vi "Perform_large_file_Analysis.vi"(7 "error in":errorcluster) -> (2 "Wvfm":waveform(dbl)[](array[waveform]), 3 "Filtered Nb of Events":i32, 5 "Total Nb of Events":dbl)   [LabVIEW 2019]
uses:
  <vilib>/Utility/error.llb/DialogType.ctl
  ESA_Data_Analysis_Global_VIs.vi
  SiPM_Tests_Global_Var.vi
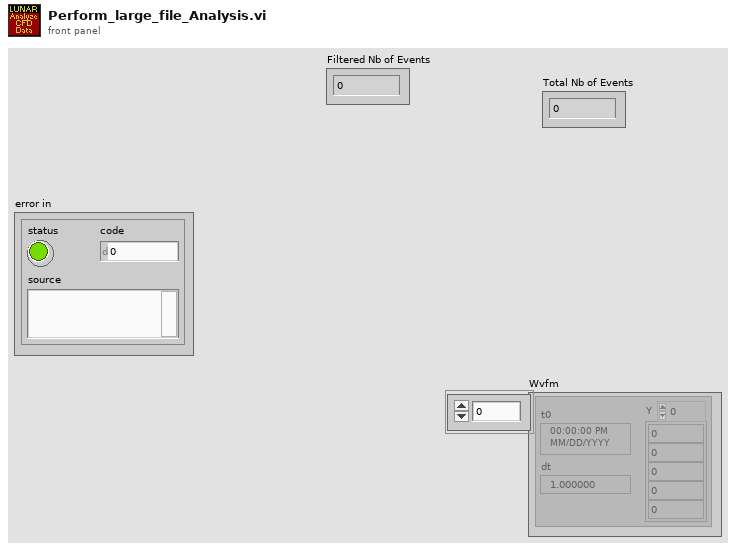
[diagram p1: front panel]
types:
  T1 = typedef "DialogType.ctl" = u16
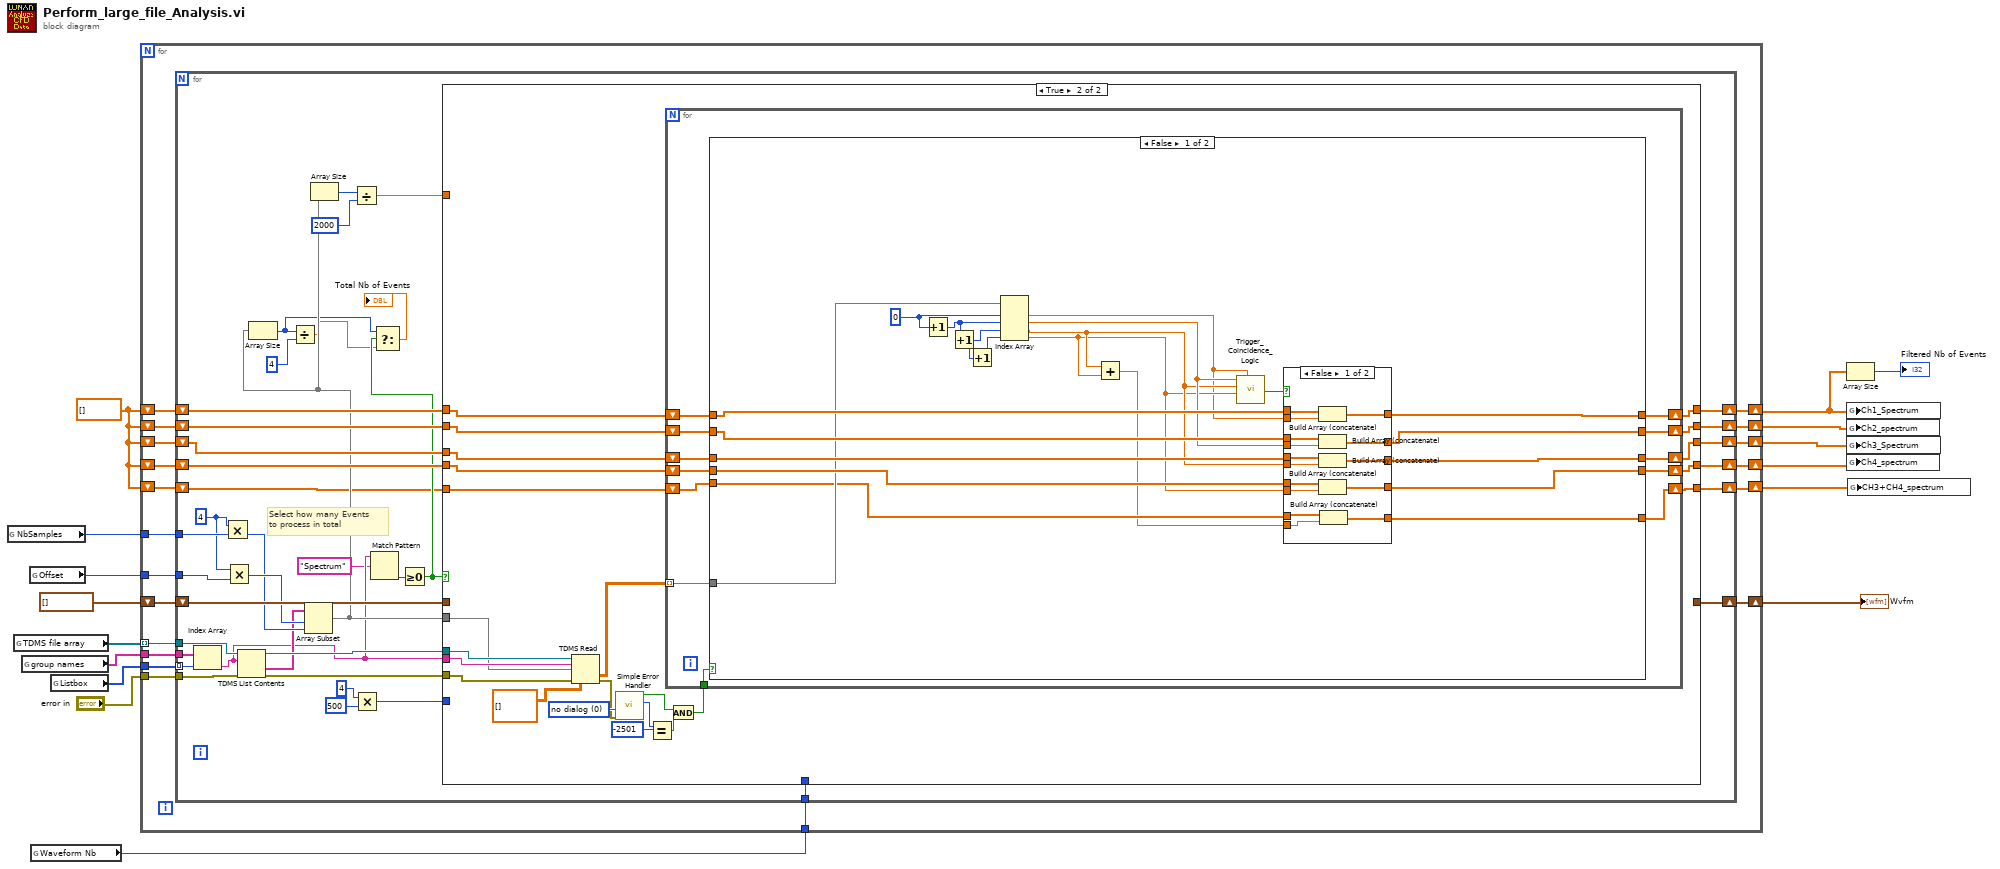
[diagram p0: block diagram]
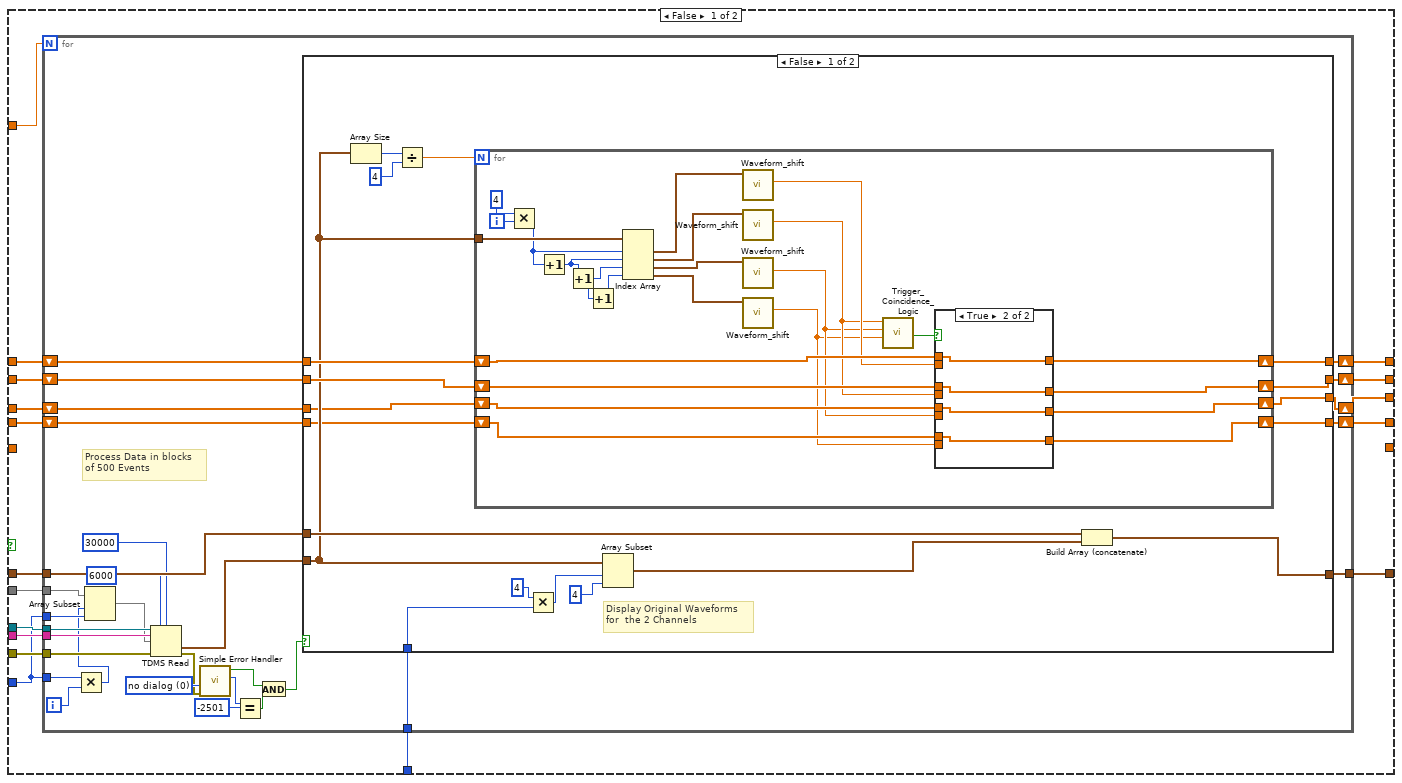
[diagram p2: hidden frame]
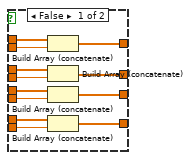
[diagram p3: hidden frame]
diagram:
  w2 = dbl[] []
  n1 = global read "SiPM_Tests_Global_Var.vi" "NbSamples"() -> (w9:i64)
  n2 = global read "SiPM_Tests_Global_Var.vi" "TDMS file array"() -> (w13:refnum<k34>[])
  n3 = global read "ESA_Data_Analysis_Global_VIs.vi" "group names"() -> (w16:string[])
  n4 = global read "SiPM_Tests_Global_Var.vi" "Offset"() -> (w11:i64)
  n5 = global read "SiPM_Tests_Global_Var.vi" "Waveform Nb"() -> (w8:u16)
  n6 = global read "ESA_Data_Analysis_Global_VIs.vi" "Listbox"() -> (w15:i32[])
  n7 = for {
    tunnel: w13 -> [w35] mode=indexing
    tunnel: w16 -> [w34]
    tunnel: w15 -> [w33]
    tunnel: "error in" -> [w32]
    tunnel: w11 -> [w30]
    shift-right: [w31] -> w12
    shift-left: waveform(dbl)[] [] -> [w29]
    shift-right: [w25] -> w7
    shift-left: w2 -> [w28]
    shift-right: [w26] -> w4
    shift-left: w2 -> [w27]
    tunnel: w9 -> [w24]
    tunnel: w8 -> [w23]
    shift-right: [w20] -> w6
    shift-left: w2 -> [w22]
    shift-right: [w19] -> w5
    shift-left: w2 -> [w21]
    shift-right: [w17] -> w1
    shift-left: w2 -> [w18]
    n8 = for {
      tunnel: w35 -> [w75]
      tunnel: w34 -> [w74]
      tunnel: w33 -> [w73] mode=indexing
      tunnel: w32 -> [w72]
      tunnel: w30 -> [w62]
      shift-right: [w69] -> w31
      shift-left: w29 -> [w68]
      shift-right: [w64] -> w25
      shift-left: w28 -> [w67]
      shift-right: [w65] -> w26
      shift-left: w27 -> [w66]
      tunnel: w24 -> [w61]
      tunnel: w23 -> [w63]
      shift-right: [w57] -> w20
      shift-left: w22 -> [w59]
      shift-right: [w56] -> w19
      shift-left: w21 -> [w58]
      shift-right: [w36] -> w17
      shift-left: w18 -> [w37]
      w60 = i64 4 ("x")
      # "Select how many Events \nto process in total"
      n9 = Index Array(array=w74, index=w73) -> (element=w44:string)
      n10 = Multiply(x=w60, y=w61) -> (x*y=w54:i64)
      n11 = Multiply(x=w60, y=w62) -> (x*y=w55:i64)
      n12 = TDMS List Contents(4:w72, 6:w44, 7:w75) -> (0:w70:errorcluster, 1:w53:string[], 3:w71:refnum<k34>)  [unwired: 1 out]
      n13 = Array Subset(array=w53, index=w55, length=w54) -> (w45:string[])
      n14 = Array Size(array=w45) -> (size(s)=w40:i32)
      n15 = Divide(x=w40, y=4) -> (x/y=w39:dbl)
      n16 = Array Size(array=w45) -> (size(s)=w48:i32)
      n17 = Divide(x=w48, y=2000) -> (x/y=w47:dbl)
      n18 = Multiply(x=i64 4, y=i64 500) -> (x*y=w50:i64)
      n19 = Match Pattern(string=w44, regular expression="Spectrum") -> (offset past match=w42:i32)  [unwired: 1 in, 3 out]
      n20 = Greater Or Equal To 0?(x=w42) -> (x >= 0?=w41:bool)
      n21 = Select(t=w40, s=w41, f=w39) -> (s? t:f=→"Total Nb of Events":dbl)
      n22 = case shown="True" w41 {
        tunnel: w71 -> [w92 w207]
        tunnel: w44 -> [w91 w208]
        tunnel: w70 -> [w90 w209]
        tunnel: [w89 _] -> w69
        tunnel: w68 -> [w88 _]
        tunnel: w67 -> [w87 w197]
        tunnel: w66 -> [w86 w198]
        tunnel: [w85 w194] -> w65
        tunnel: [w84 w193] -> w64
        tunnel: w63 -> [w83 _]
        tunnel: w59 -> [w82 w196]
        tunnel: w58 -> [w81 w195]
        tunnel: [w80 w192] -> w57
        tunnel: [w79 w191] -> w56
        tunnel: w50 -> [w78 _]
        tunnel: w47 -> [w77 _]
        tunnel: w45 -> [w76 w190]
        tunnel: w37 -> [_ w188]
        tunnel: [_ w187] -> w36
        frame False {
          n23 = for {
            N: w77 -> [_]
            tunnel: w92 -> [w122]
            tunnel: w91 -> [w121]
            tunnel: w90 -> [w118]
            tunnel: [w117] -> w89
            tunnel: w88 -> [w116]
            tunnel: w83 -> [w106]
            tunnel: w76 -> [w100]
            shift-right: [w108] -> w85
            shift-left: w86 -> [w109]
            shift-right: [w107] -> w84
            shift-left: w87 -> [w110]
            shift-right: [w103] -> w80
            shift-left: w82 -> [w105]
            shift-right: [w102] -> w79
            shift-left: w81 -> [w104]
            tunnel: w78 -> [w98]
            tunnel: w78 -> [w96]
            i -> [w97]
            w120 = T1 0 items=["no dialog", "OK message", "continue or stop message", "OK message + warnings", "continue/stop + warnings"] ("type of dialog (OK msg:1)")
            # "Process Data in blocks \nof 500 Events"
            n24 = Multiply(x=w96, y=w97) -> (x*y=w95:i64)
            n25 = Array Subset(array=w100, index=w95, length=w98) -> (w99:string[])
            n26 = TDMS Read(0:w122, 1:i64 6000 ("offset (0)"), 2:i64 30000 ("count (-1: all)"), 5:w121, 7:w99, 11:w118) -> (10:w101:waveform(dbl)[], 15:w119:errorcluster)  [unwired: 2 in, 4 out]
            n27 = call <vilib>:"Simple Error Handler.vi"("type of dialog (OK msg:1)"=w120, "error in (no error)"=w119) -> ("error?"=w114:bool, "code out"=w113:i32)  [unwired: 3 in, 3 out]
            n28 = Equal?(x=w113, y=-2501) -> (x = y?=w111:bool)
            n29 = And(x=w114, y=w111) -> (x .and. y?=w115:bool)
            n30 = case shown="False" w115 {
              tunnel: w101 -> [w127 _]
              tunnel: [w140 w186] -> w117
              tunnel: w116 -> [w139 w186]
              tunnel: w110 -> [w135 w184]
              tunnel: w109 -> [w134 w185]
              tunnel: [w133 w185] -> w108
              tunnel: [w132 w184] -> w107
              tunnel: w106 -> [w128 _]
              tunnel: w105 -> [w126 w183]
              tunnel: w104 -> [w125 w182]
              tunnel: [w124 w183] -> w103
              tunnel: [w123 w182] -> w102
              frame False {
                # "Display Original Waveforms\nfor  the 2 Channels"
                n31 = Array Size(array=w127) -> (size(s)=w138:i32)
                n32 = Divide(x=w138, y=4) -> (x/y=w136:dbl)
                n33 = for {
                  N: w136 -> [_]
                  tunnel: w127 -> [w165]
                  shift-right: [w152] -> w133
                  shift-left: w134 -> [w153]
                  shift-right: [w150] -> w132
                  shift-left: w135 -> [w160]
                  shift-right: [w148] -> w124
                  shift-left: w126 -> [w149]
                  shift-right: [w147] -> w123
                  shift-left: w125 -> [w146]
                  i -> [w159]
                  n34 = Multiply(x=4, y=w159) -> (x*y=w163:i32)
                  n35 = Increment(x=w163) -> (x+1=w158:i32)
                  n36 = Increment(x=w158) -> (x+1=w156:i32)
                  n37 = Increment(x=w156) -> (x+1=w157:i32)
                  n38 = Index Array(array=w165, index #1=w163, index #2=w158, index #3=w156, index #4=w157) -> (element #1=w162:waveform(dbl), element #2=w161:waveform(dbl), element #3=w155:waveform(dbl), element #4=w154:waveform(dbl))
                  n39 = call "Waveform_shift.vi"("Waveform_in"=w162) -> ("Peak Value"=w151:dbl)  [unwired: 9 in]
                  n40 = call "Waveform_shift.vi"("Waveform_in"=w161) -> ("Peak Value"=w144:dbl)  [unwired: 9 in]
                  n41 = call "Waveform_shift.vi"("Waveform_in"=w155) -> ("Peak Value"=w143:dbl)  [unwired: 9 in]
                  n42 = call "Waveform_shift.vi"("Waveform_in"=w154) -> ("Peak Value"=w142:dbl)  [unwired: 9 in]
                  n43 = call "Trigger_Coincidence_Logic.vi"("Peak_ch4"=w142, "Peak_ch3"=w143, "Peak_ch2"=w144) -> ("Filter-out"=w145:bool)  [unwired: 8 in]
                  n44 = case shown="True" w145 {
                    tunnel: w160 -> [w177 w180]
                    tunnel: w144 -> [w176 _]
                    tunnel: w153 -> [w175 w181]
                    tunnel: [w174 w181] -> w152
                    tunnel: w151 -> [w173 _]
                    tunnel: [w172 w180] -> w150
                    tunnel: w149 -> [w171 w179]
                    tunnel: w143 -> [w170 _]
                    tunnel: [w169 w179] -> w148
                    tunnel: [w168 w178] -> w147
                    tunnel: w146 -> [w167 w178]
                    tunnel: w142 -> [w166 _]
                    frame False {
                      n45 = Build Array (concatenate)(w175, w173) -> (w174:dbl[])
                      n46 = Build Array (concatenate)(w177, w176) -> (w172:dbl[])
                      n47 = Build Array (concatenate)(w171, w170) -> (w169:dbl[])
                      n48 = Build Array (concatenate)(w167, w166) -> (w168:dbl[])
                    }
                    frame True {
                    }
                  }
                }
                n49 = Multiply(x=4, y=w128) -> (x*y=w131:i32)
                n50 = Array Subset(array=w127, index=w131, length=4) -> (w141:waveform(dbl)[])
                n51 = Build Array (concatenate)(w139, w141) -> (w140:waveform(dbl)[])
              }
              frame True {
              }
            }
          }
        }
        frame True {
          w206 = T1 0 items=["no dialog", "OK message", "continue or stop message", "OK message + warnings", "continue/stop + warnings"] ("type of dialog (OK msg:1)")
          n52 = TDMS Read(0:w207, 5:w208, 7:w190, 11:w209, 12:dbl[][] []) -> (10:w199:dbl[][], 15:w205:errorcluster)  [unwired: 3 in, 4 out]
          n53 = call <vilib>:"Simple Error Handler.vi"("type of dialog (OK msg:1)"=w206, "error in (no error)"=w205) -> ("error?"=w203:bool, "code out"=w202:i32)  [unwired: 3 in, 3 out]
          n54 = Equal?(x=w202, y=-2501) -> (x = y?=w200:bool)
          n55 = And(x=w203, y=w200) -> (x .and. y?=w204:bool)
          n56 = for {
            tunnel: w204 -> [w221]
            tunnel: w199 -> [w220] mode=indexing
            shift-right: [w212] -> w191
            shift-left: w195 -> [w216]
            shift-right: [w213] -> w192
            shift-left: w196 -> [w217]
            shift-right: [w214] -> w193
            shift-left: w197 -> [w218]
            shift-right: [w215] -> w194
            shift-left: w198 -> [w219]
            shift-right: [w210] -> w187
            shift-left: w188 -> [w211]
            n57 = case shown="False" w221 {
              tunnel: w218 -> [w242 w266]
              tunnel: w219 -> [w241 w267]
              tunnel: [w240 w267] -> w215
              tunnel: [w239 w266] -> w214
              tunnel: w217 -> [w238 w265]
              tunnel: w216 -> [w237 w264]
              tunnel: [w236 w265] -> w213
              tunnel: [w235 w264] -> w212
              tunnel: w220 -> [w234 _]
              tunnel: w211 -> [w225 w263]
              tunnel: [w223 w263] -> w210
              frame False {
                w228 = 0 ("x")
                n58 = Increment(x=w228) -> (x+1=w233:i32)
                n59 = Increment(x=w233) -> (x+1=w231:i32)
                n60 = Increment(x=w231) -> (x+1=w232:i32)
                n61 = Index Array(array=w234, index #1=w228, index #2=w233, index #3=w231, index #4=w232) -> (element #1=w222:dbl, element #2=w229:dbl, element #3=w227:dbl, element #4=w226:dbl)
                n62 = Add(x=w227, y=w226) -> (x+y=w224:dbl)
                n63 = call "Trigger_Coincidence_Logic.vi"("Peak_ch1"=w222, "Peak_ch4"=w226, "Peak_ch3"=w227, "Peak_ch2"=w229) -> ("Filter-out"=w230:bool)  [unwired: 7 in]
                n64 = case shown="False" w230 {
                  tunnel: w242 -> [w257 w261]
                  tunnel: w229 -> [w256 _]
                  tunnel: w241 -> [w255 w262]
                  tunnel: [w254 w262] -> w240
                  tunnel: w222 -> [w253 _]
                  tunnel: [w252 w261] -> w239
                  tunnel: w238 -> [w251 w260]
                  tunnel: w227 -> [w250 _]
                  tunnel: [w249 w260] -> w236
                  tunnel: [w248 w259] -> w235
                  tunnel: w237 -> [w247 w259]
                  tunnel: w226 -> [w246 _]
                  tunnel: w225 -> [w245 w258]
                  tunnel: w224 -> [w244 _]
                  tunnel: [w243 w258] -> w223
                  frame False {
                    n65 = Build Array (concatenate)(w255, w253) -> (w254:dbl[])
                    n66 = Build Array (concatenate)(w257, w256) -> (w252:dbl[])
                    n67 = Build Array (concatenate)(w251, w250) -> (w249:dbl[])
                    n68 = Build Array (concatenate)(w247, w246) -> (w248:dbl[])
                    n69 = Build Array (concatenate)(w245, w244) -> (w243:dbl[])
                  }
                  frame True {
                  }
                }
              }
              frame True {
              }
            }
          }
        }
      }
    }
  }
  "Wvfm" <- w12
  n70 = Array Size(array=w4) -> (size(s)=→"Filtered Nb of Events":i32)
  n71 = global write "SiPM_Tests_Global_Var.vi" "Ch1_Spectrum"(w4) -> ()
  n72 = global write "SiPM_Tests_Global_Var.vi" "Ch2_spectrum"(w7) -> ()
  n73 = global write "SiPM_Tests_Global_Var.vi" "Ch3_Spectrum"(w6) -> ()
  n74 = global write "SiPM_Tests_Global_Var.vi" "Ch4_spectrum"(w5) -> ()
  n75 = global write "SiPM_Tests_Global_Var.vi" "CH3+CH4_spectrum"(w1) -> ()
